vi "LEBITVacuum.SetSafety.vi"(0 "i ref in":refnum<vi>, 2 "index of element":i32, 3 "Set Value":i16, 4 "Safety Value":i16, 5 "error IO":errorcluster) -> (14 "i ref out":refnum<vi>, 19 "error out":errorcluster)   [LabVIEW 2014, in "LEBITVacuum.lvlib"]
uses:
  LEBITVacuum.lvlib
  CS_Core/CSSystem/CoreDefs/CoreDefs.error_type.ctl
  CS_Core/CSSystem/CoreDefs/CoreDefs.error_severity.ctl
  CS_Core/CSSystem/CoreLib/CoreLib.lvlib
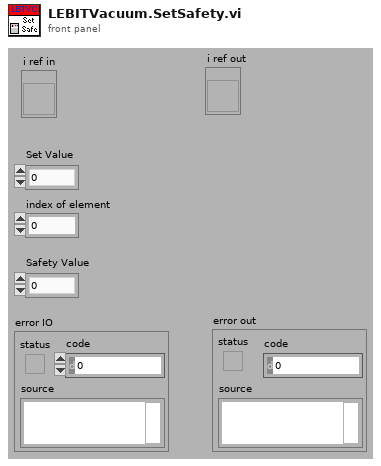
[diagram p1: front panel]
types:
  T1 = typedef "CoreDefs.error_severity.ctl" = enum16{"undefined", "information", "warning", "error", "fatal"}
  T2 = typedef "CoreDefs.error_type.ctl" = enum16{"no error", "can't load process", "can't unload process", "process does not exist", "can't install process", "can't remove process", "unknown function", "time out", "can't execute function", "duplicate queue name", "super not found", "caller queue invalid", "can't ping process", "unknown error", "VISA Error", "VISA timeout", "GPIB timeout", "GPIB error", "communication error", "data type mismatch", "can't read data from OPC server", "can't write data to OPC server", "OET error", "function not implemented", "process already exists", "invalid Shared Variable name", "error writing Shared Variable", "error reading Shared Variable", "invalid client name", "corrupt database", "unknown class", "call not authorized", "parameter out of range", "OET timeout: can't get data to modify", "invalid queue name", "requested operation incompatible with current state", "event undefined", "event disabled", "state undefined", "caller is not a friend", "EventBuilder: bad eventID", "EventBuilder: no DAQ devices", "a thread must not stop itself", "UNUSED ELEMENT4", "DiscArchiver: eventData incomplete", "DiscArchiver: eventData does not belong to run", "DiscArchiver: can't open file", "DiscArchiver: can't write to file", "DiscArchiver: available disc space low", "can't acquire semaphore", "error reading data from database", "notifier object is not existing", "can't register process", "can't unregister process", "illegal event type", "object disabled", "object already exists", "can't change state", "Instrument not found", "no connection to remote node", "invalid reference", "N/A", "UNUSED ELEMENT 1", "element not found", "illegal TCP/IP connection detected", "object does not exist", "invalid access ID", "unknown CS system", "invalid privilige", "unsupported data type", "unsupported server type", "IO server already exists", "Shared Variable already exists"}
  T3 = typedef "LEBITVacuum.lvlib/LEBITVacuum.i attribute.ctl" = cluster{"setValuePLC":string[], "nickNames":string[], "setValuePLCServiceID":i32[], "monValuePLC":string[], "SetValueServiceID":i32[], "MonValueServiceID":i32[], "SetValue":i16[], "AllPLCValues":string[], "CondSpecial2DArray":string[][], "CondSpecialIndex":i32[], "ReasonForLocking":string, "ReasonForLockingID":i32, "enableValuePLC":string[], "OverwriteCloseSafetyPLC":string[], "OverwriteOpenSafetyPLC":string[], "OverwriteCloseSafetyPLCServiceID":i32[], "OverwriteOpenSafetyPLCServiceID":i32[], "MKS Address Array":i32[][], "MKS MeasurementServiceID":i32[], "MKS Measurement":string[], "CRYO Measurement":string[][], "CRYO MeasurementServiceID":i32[], "Special":string[], "Start Date":string, "MKS VISA resource":refnum<visa-resource-name>, "CRYO VISA resource":refnum<visa-resource-name>}
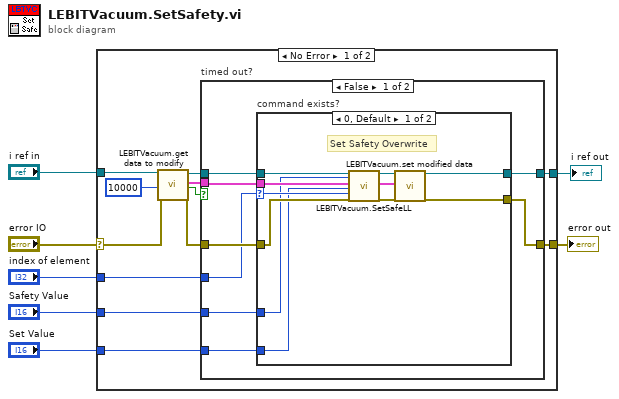
[diagram p0: block diagram]
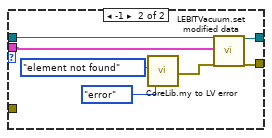
[diagram p2: hidden frame]
diagram:
  n1 = case shown="No Error" "error IO" {
    selector: "error IO" -> [w14 w48]
    tunnel: "i ref in" -> [w17 w49]
    tunnel: [w16 w48] -> w6
    tunnel: [w15 w49] -> w5
    tunnel: "Set Value" -> [w10 _]
    tunnel: "index of element" -> [w9 _]
    tunnel: "Safety Value" -> [w8 _]
    frame No Error {
      n2 = call "LEBITVacuum.get data to modify.vi"("i ref in"=w17, "ms timeout (10000)"=10000, "error in (no error)"=w14) -> ("i ref out"=w18:refnum<vi>, "i attribute"=w19:T3, "timed out"=w12:bool, "error out"=w11:errorcluster)  [unwired: 13 in]
      n3 = case "timed out?" shown="False" w12 {
        tunnel: w19 -> [w27 _]
        tunnel: w18 -> [w26 w47]
        tunnel: [w24 w46] -> w16
        tunnel: [w23 w47] -> w15
        tunnel: w11 -> [w25 w46]
        tunnel: w10 -> [w22 _]
        tunnel: w9 -> [w21 _]
        tunnel: w8 -> [w20 _]
        frame False {
          n4 = case "command exists?" shown="0, Default" w21 {
            selector: w21 -> [w33 _]
            tunnel: [w37 w42] -> w23
            tunnel: [w38 w39] -> w24
            tunnel: w26 -> [w36 w43]
            tunnel: w27 -> [w35 w41]
            tunnel: w25 -> [w34 _]
            tunnel: w22 -> [w32 _]
            tunnel: w20 -> [w28 _]
            frame 0, Default {
              # "Set Safety Overwrite"
              n5 = call "LEBITVacuum.SetSafeLL.vi"("i ref in"=w36, "Set Safety"=w28, "i attribute in"=w35, "SetValue"=w32, "index of element"=w33, "error IO"=w34) -> ("i ref out"=w31:refnum<vi>, "i attribute out"=w30:T3, "error out"=w29:errorcluster)  [unwired: 11 in]
              n6 = call "LEBITVacuum.set modified data.vi"("i ref in"=w31, "i attribute"=w30, "error in (no error)"=w29) -> ("i ref out"=w37:refnum<vi>, "error out"=w38:errorcluster)  [unwired: 15 in]
            }
            frame -1 {
              n7 = call "CoreLib.my to LV error.vi"("ErrorTypes"=CoreDefs.error_type."element not found", "severityLevel"=CoreDefs.error_severity."error") -> ("myErrorCluster"=w40:errorcluster)  [unwired: 16 in, 1 out]
              n8 = call "LEBITVacuum.set modified data.vi"("i ref in"=w43, "i attribute"=w41, "error in (no error)"=w40) -> ("i ref out"=w42:refnum<vi>, "error out"=w39:errorcluster)  [unwired: 15 in]
            }
          }
        }
        frame True {
        }
      }
    }
    frame Error {
    }
  }
  "error out" <- w6
  "i ref out" <- w5
